vi "LVObject to JSON - Inline Type Name Handling - Output Is Pretty Printed.vi"() -> ()   [LabVIEW 2017, in "Generic Object Serializer Tests.lvlib" / "Pretty Print.lvlib"]
uses:
  Pretty Print.lvlib
  Generic Object Serializer/Generic Object Serializer.lvclass
  Generic Object Serializer/Type Name Handling.ctl
  Generic Object Serializer/Generic Object Serializer.lvclass/Generic Object Serializer.ctl
  Generic Object Serializer/Write Type Name Handling.vi
  <vilib>/addons/_JKI Toolkits/Caraya/classes/Assert/Assert Equal Value_Variant.vi
  <vilib>/addons/_JKI Toolkits/Caraya/classes/Test/Test.lvclass
  <vilib>/addons/_JKI Toolkits/Caraya/classes/Assert/Assert.lvclass
  Temperature Forecast/Temperature Forecast.lvclass
panel:
  out "error out":errorcluster
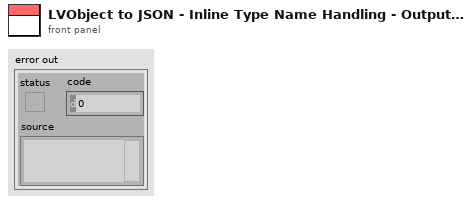
[diagram p1: front panel]
types:
  T1 = typedef "Generic Object Serializer.lvclass/Type Name Handling.ctl" = enum16{"None", "Inline"}
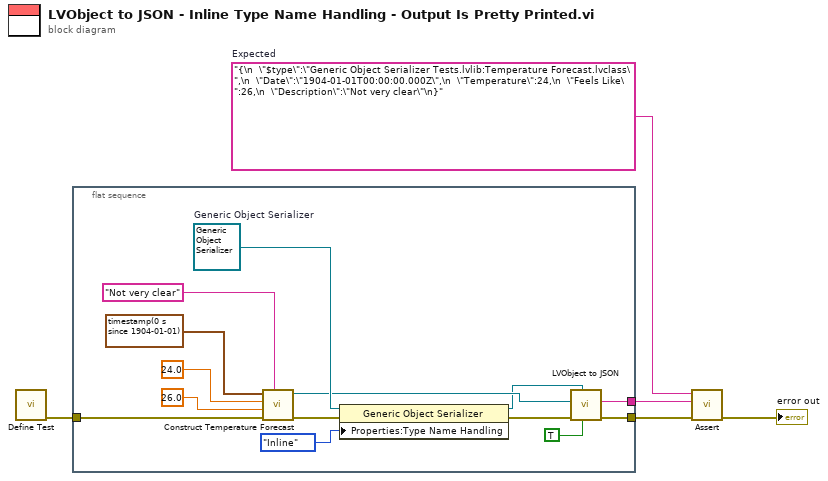
[diagram p0: block diagram]
diagram:
  w1 = "{\n  \"$type\":\"Generic Object Serializer Tests.lvlib:Temperature Forecast.lvclass\",\n  \"Date\":\"1904-01-01T00:00:00.000Z\",\n  \"Temperature\":24,\n  \"Feels Like\":26,\n  \"Description\":\"Not very clear\"\n}"  # Expected
  n1 = call <vilib>:"Define Test.vi"() -> ("error out"=w4:errorcluster)  [unwired: 11 in]
  n2 = flat-sequence {
    tunnel: w4 -> [w12]
    tunnel: [w18] -> w3
    tunnel: [w17] -> w2
    frame #0 {
      w19 = refnum<class "Generic Object Serializer.lvclass"> refnum  # Generic Object Serializer
      n3 = call "Construct Temperature Forecast.vi"("Description"="Not very clear", "error in (no error)"=w12, "Feels Like [°C]"=26.0, "Temperature [°C]"=24.0, "Date"=timestamp(0 s since 1904-01-01)) -> ("error out"=w7:errorcluster, "Temperature Forecast"=w11:refnum<class "Temperature Forecast.lvclass">)  [unwired: 5 in]
      n4 = property class="Generic Object Serializer"(reference=w19, error in=w7, "Properties:Type Name Handling"=Type_Name_Handling."Inline" ("Type Name Handling")) -> (reference out=w9:refnum<class "Generic Object Serializer.lvclass">, error out=w6:errorcluster)
      n5 = call-dynamic "LVObject to JSON.vi"("Pretty Print?"=TRUE, "LVClass Serializer"=w9, "error in (no error)"=w6, "Object"=w11) -> ("error out"=w18:errorcluster, "<JSON>Object"=w17:string)  [unwired: 6 in]
    }
  }
  n6 = call-poly <vilib>:"Assert.vi"("error in (no error)"=w3, "Y"=w2, "X"=w1) -> ("error out"=→"error out":errorcluster)  [unwired: 8 in]
